vi "Testing DB Query.vi"() -> ()   [LabVIEW 2009]
uses:
  Controls/ALTS Station Details.ctl
  Controls/Status Ring Indicator v1.ctl
  Controls/ALTS Obtain Test Data DB Driver Options.ctl
  Controls/ALTS Station Cluster.ctl
  <vilib>/addons/database/Recordset.llb/Rec Destroy - Connection.vi
  <vilib>/addons/database/Recordset.llb/Rec Fetch Recordset Data (R).vi
  <vilib>/addons/database/Connection.llb/Conn Execute.vi
  <vilib>/addons/database/Connection.llb/DB Tools Open Connec (Path).vi
  <vilib>/addons/database/NI_Database_API.lvlib
panel:
  in  "Station Cluster 2":T1
  out "Station Cluster":T1
  out "data 2":string[][](array[string])
  out "error out 2":errorcluster
  in  "error in":errorcluster
  out "error out":errorcluster
  in  "connection information":path
  out "data":string[][](array[string])
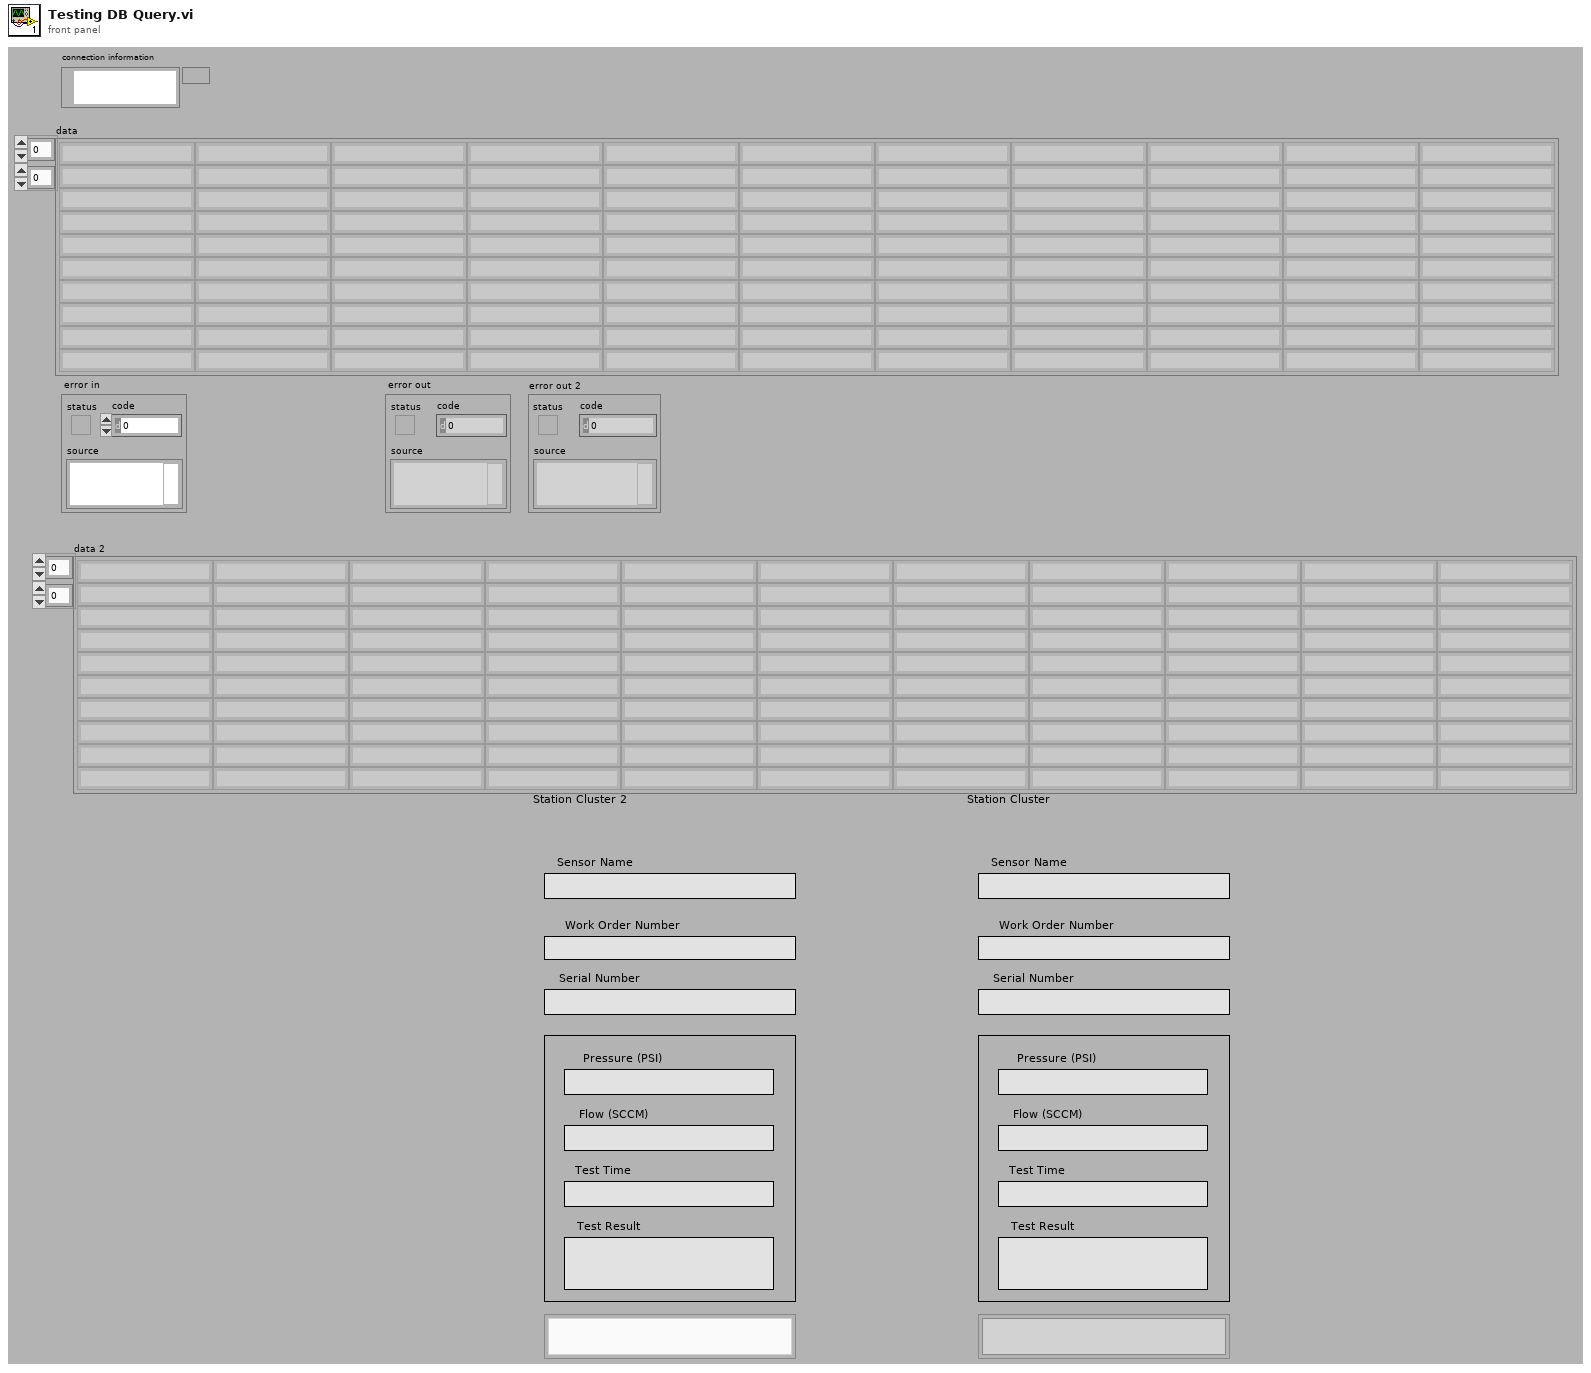
[diagram p1: front panel]
types:
  T1 = typedef "ALTS Station Details.ctl" = cluster{"Station Number":string, "Work Order Number":string, "Sensor Name":string, "Pressure (PSI)":string, "Flow (SCCM)":string, "Test Time ":string, "Test Result":string, "Station Status":T2, "Serial Number":string}
  T2 = typedef "Status Ring Indicator v1.ctl" = u16
  T3 = typedef "ALTS Station Cluster.ctl" = enum16{"Station 1", "Station 2", "Station 3", "Station 4"}
  T4 = typedef "ALTS Obtain Test Data DB Driver Options.ctl" = enum16{"Init", "Read Test Data Results", "Close"}
  T5 = typedef "NI_Database_API.lvlib/Conn ObjectReference.ctl" = refnum<k1>
  T6 = typedef "NI_Database_API.lvlib/Rec ObjectReference.ctl" = refnum<k1>
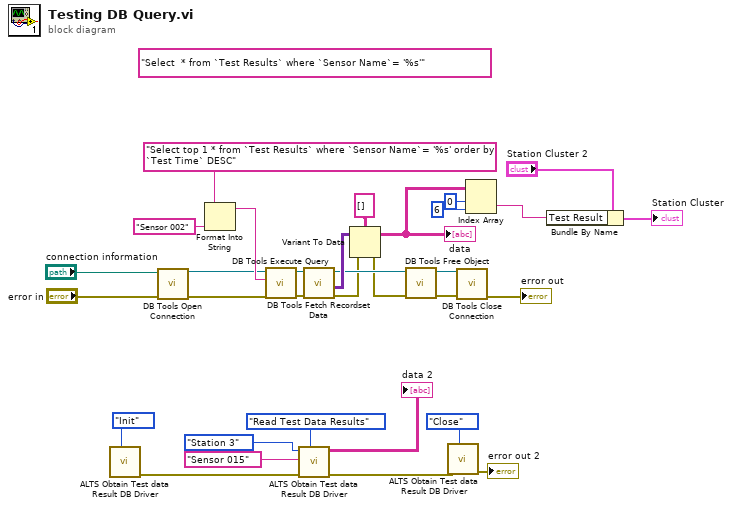
[diagram p0: block diagram]
diagram:
  (unwired) "Select  * from `Test Results` where `Sensor Name`= '%s'" ("format string")
  n1 = call "ALTS Obtain Test data Result DB Driver.vi"("Option"=ALTS_Obtain_Test_Data_DB_Driver_Options."Init") -> ("error out"=w12:errorcluster)  [unwired: 9 in, 1 out]
  n2 = call-poly <vilib>:"DB Tools Open Connection.vi"("error in (no error)"="error in", "connection information"="connection information") -> ("error out"=w23:errorcluster, "connection reference"=w24:T5)  [unwired: 6 in]
  n3 = Format Into String(format string="Select top 1 * from `Test Results` where `Sensor Name`= '%s' order by `Test Time` DESC", "Sensor 002" ("input 1")) -> (resulting string=w25:string)  [unwired: 2 in, 1 out]
  n4 = call-poly <vilib>:"DB Tools Execute Query.vi"("error in (no error)"=w23, "SQL query"=w25, "connection reference"=w24) -> ("error out"=w27:errorcluster, "recordset reference"=w26:T6)  [unwired: 5 in]
  n5 = call "ALTS Obtain Test data Result DB Driver.vi"("Option"=ALTS_Obtain_Test_Data_DB_Driver_Options."Read Test Data Results", "error in"=w12, "Sensor Name"="Sensor 015" ("input 1"), "Station Enum"=ALTS_Station_Cluster."Station 3") -> ("error out"=w13:errorcluster, "data"=→"data 2":string[][])  [unwired: 6 in]
  n6 = call-poly <vilib>:"DB Tools Fetch Recordset Data.vi"("error in (no error)"=w27, "recordset reference"=w26) -> ("error out"=w29:errorcluster, "recordset data"=w32:variant[][], "recordset reference out"=w31:T6)  [unwired: 3 in]
  n7 = Variant To Data(error in=w29, Variant=w32, type=string[][] []) -> (error out=w30:errorcluster, data=w5:string[][])
  "data" <- w5
  n8 = call-poly <vilib>:"DB Tools Free Object.vi"("error in (no error)"=w30, "recordset reference"=w31) -> ("error out"=w20:errorcluster, "connection reference"=w21:T5)  [unwired: 8 in]
  n9 = call "ALTS Obtain Test data Result DB Driver.vi"("Option"=ALTS_Obtain_Test_Data_DB_Driver_Options."Close", "error in"=w13) -> ("error out"=→"error out 2":errorcluster)  [unwired: 8 in, 1 out]
  n10 = call <vilib>:"DB Tools Close Connection.vi"("error in (no error)"=w20, "connection reference"=w21) -> ("error out"=→"error out":errorcluster)  [unwired: 5 in]
  n11 = Index Array(array=w5, index (row)=0, index (col)=6 ("disabled index (col)")) -> (element=w2:string)
  n12 = Bundle By Name(cluster="Station Cluster 2", "Test Result"=w2) -> (→"Station Cluster":T1)
